vi "Get Endpoints.vi"(8 "error in (no error)":errorcluster, 11 "Manager in":refnum<class "Manager.lvclass">) -> (0 "error out":errorcluster, 2 "Endpoints":refnum<class "Endpoint.lvclass">[](array[class]), 3 "Manager out":refnum<class "Manager.lvclass">)   [LabVIEW 2020, in "Stream-Simple-Msg.lvlib" / "Manager.lvclass"]
uses:
  Manager.lvclass
  Endpoint/Endpoint.lvclass
  Manager.lvclass/Manager.ctl
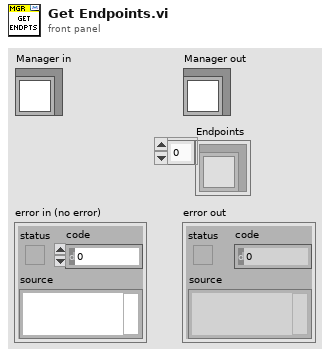
[diagram p1: front panel]
types:
  T1 = typedef "Stream-Simple-Msg.lvlib/Manager.lvclass/Ref Data.ctl" = cluster{"Message Callbacks":map{string, T2[]}, "Endpoints":map{string, refnum<class "Endpoint.lvclass">}, "Stream Endpoints":refnum<class "Endpoint.lvclass">[]}
  T2 = typedef "Stream-Simple-Msg.lvlib/Manager.lvclass/Callback.ctl" = cluster{"VI":refnum<vi>, "Owner":refnum<class>}
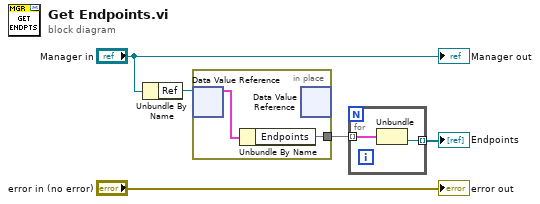
[diagram p0: block diagram]
diagram:
  n1 = Unbundle By Name("Manager in") -> ("Ref"=w3:refnum<data-value>)
  n2 = in-place {
    in-place-border: [w6] -> w2
    n3 = in-place-dvr #1(w3) -> (w7:T1)  [unwired: 1 out]
    n4 = Unbundle By Name(w7) -> ("Endpoints"=w6:map{string, refnum<class "Endpoint.lvclass">})
    n5 = in-place-dvr #1() -> ()  [unwired: 1 in, 2 out]
  }
  n6 = for {
    tunnel: w2 -> [w9] mode=indexing
    tunnel: [w8] -> w1 mode=indexing
    n7 = Unbundle(w9) -> ("Stream-Simple-Msg:Endpoint"=w8:refnum<class "Endpoint.lvclass">)  [unwired: 1 out]
  }
  "Endpoints" <- w1
  "error out" <- "error in (no error)"
  "Manager out" <- "Manager in"
